vi "Write Data to File.vi"(4 "error in (no error)":errorcluster, 6 "Data to Write":string, 7 "File to Write":path) -> (0 "error out":errorcluster)   [LabVIEW 2011]
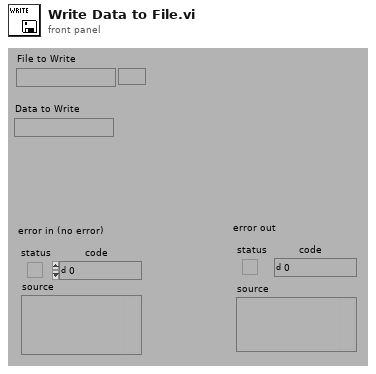
[diagram p1: front panel]
types:
  T1 = enum16{"open", "open or create", "create or replace", "create", "open (read only)"}
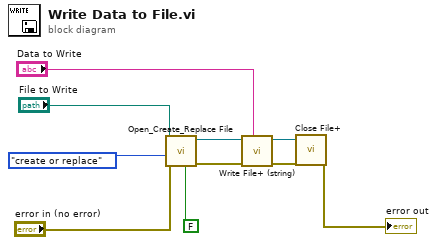
[diagram p0: block diagram]
diagram:
  n1 = call <vilib>:"Open_Create_Replace File.vi"("advisory dialog? (display:T)"=FALSE, "error in (no error)"="error in (no error)", "function (open:0)"=T1."create or replace", "file path"="File to Write") -> ("error out"=w5:errorcluster, "refnum"=w8:refnum<file>)  [unwired: 3 in, 3 out]
  n2 = call <vilib>:"Write File+ (string).vi"("string"="Data to Write", "error in (no error)"=w5, "refnum"=w8) -> ("error out"=w6:errorcluster, "dup refnum"=w7:refnum<file>)  [unwired: 2 in, 3 out]
  n3 = call <vilib>:"Close File+.vi"("error in (no error)"=w6, "refnum"=w7) -> ("error out"=→"error out":errorcluster)  [unwired: 5 out]
